vi "async send error to engine.vi"(7 "force send?":bool, 8 "command error in":errorcluster, 9 "module error":errorcluster, 10 "error classification":T1, 11 "error fifo":refnum<k33>) -> (0 "command error out":errorcluster)   [LabVIEW 2013, in "async executor.lvlib"]
uses:
  async executor/async executor.lvlib
  async error info.ctl
  <vilib>/NI/Tag Bus Module Framework/runtime/error classification.ctl
  <vilib>/NI/Tag Bus Module Framework/runtime/TBM module execution interface.lvclass
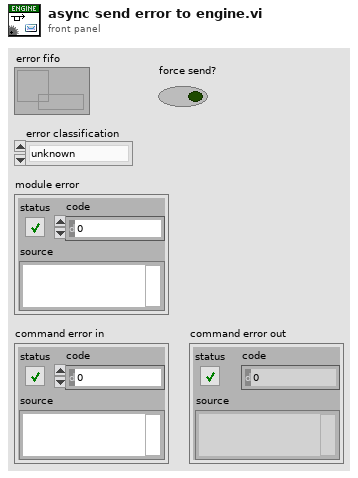
[diagram p1: front panel]
types:
  T1 = typedef "TBM module execution interface.lvclass/error classification.ctl" = enum16{"unknown", "none", "trivial", "recoverable", "critical"}
  T2 = typedef "async executor.lvlib/async error info.ctl" = cluster{"error code":i32, "error classification":T1}
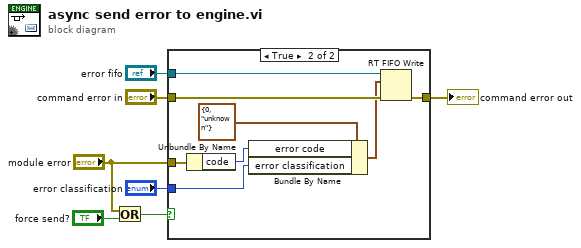
[diagram p0: block diagram]
diagram:
  n1 = Or(x="module error", y="force send?") -> (x .or. y?=w3:bool)
  n2 = case shown="True" w3 {
    tunnel: [w8 w16] -> w7
    tunnel: "command error in" -> [w8 w15]
    tunnel: "error fifo" -> [_ w14]
    tunnel: "error classification" -> [_ w10]
    tunnel: "module error" -> [_ w9]
    frame False {
    }
    frame True {
      n3 = Unbundle By Name(w9) -> ("code"=w11:i32)
      n4 = Bundle By Name(cluster=T2 {"error code"=0, "error classification"=enum."unknown"} ("element"), "error code"=w11, "error classification"=w10) -> (w12:T2)
      n5 = RT FIFO Write(0:w14, 1:w12, 3:w15) -> (11:w16:errorcluster)  [unwired: 2 in, 3 out]
    }
  }
  "command error out" <- w7
